vi "hanfei_OFDM_modulator.vi"(4 "error in (no error)":errorcluster, 5 "OFDM Parameters":T1={"FFT size (N)"=64, "Length of CP (Lc)"=8, "Null Tones"=[0, 30, 31, 32], "Training Sequence FFT size"=0, "Training Sequence Length of CP"=0, "Number of OFDM symbols (derived)"=1}, 7 "input symbols":cdb[](array[numeric])) -> (0 "error out":errorcluster, 1 "OFDM Parameters out":T1={"FFT size (N)"=64, "Length of CP (Lc)"=8, "Null Tones"=[0, 30, 31, 32], "Training Sequence FFT size"=0, "Training Sequence Length of CP"=0, "Number of OFDM symbols (derived)"=1}, 3 "output samples":cdb[](array[numeric]))   [LabVIEW 2015]
uses:
  OFDM_parameters.ctl
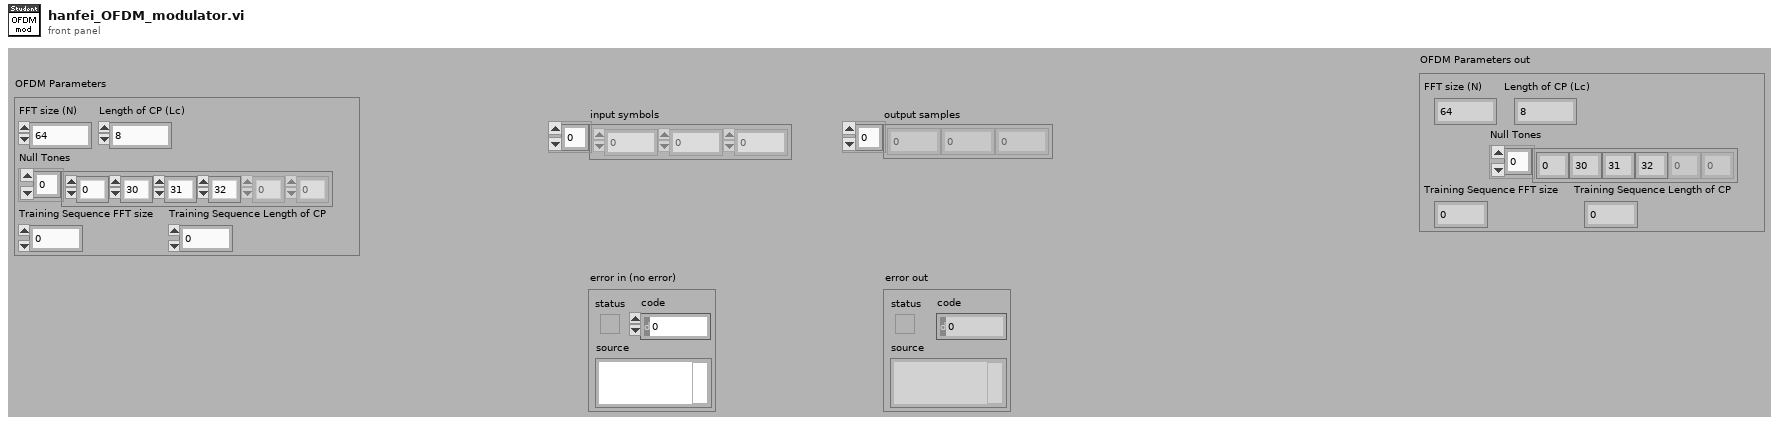
[diagram p1: front panel]
types:
  T1 = typedef "OFDM_parameters.ctl" = cluster{"FFT size (N)":i32, "Length of CP (Lc)":i32, "Null Tones":u32[], "Training Sequence FFT size":i32, "Training Sequence Length of CP":i32, "Number of OFDM symbols (derived)":i32}
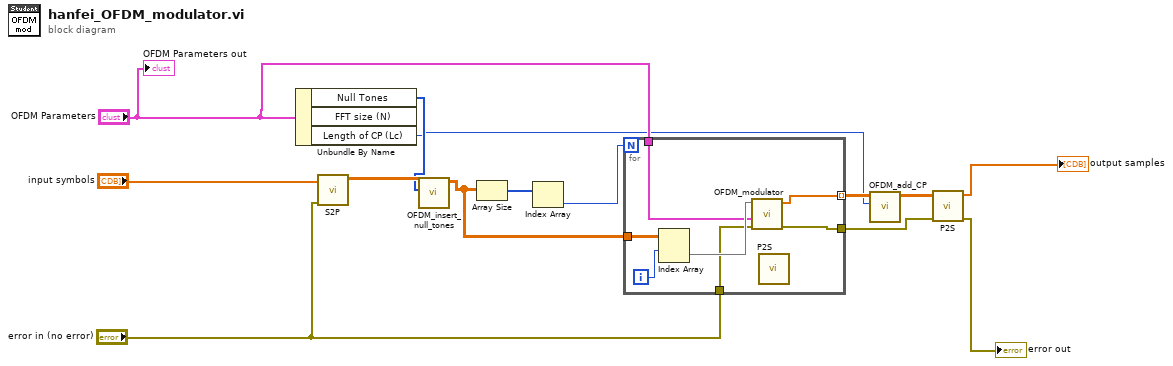
[diagram p0: block diagram]
diagram:
  n1 = Unbundle By Name("OFDM Parameters") -> ("Null Tones"=w12:u32[], "Length of CP (Lc)"=w1:i32)  [unwired: 1 out]
  n2 = call "S2P.vi"("error in (no error)"="error in (no error)", "serial input"="input symbols") -> ("parallel output"=w13:cdb[][])  [unwired: 4 in, 1 out]
  n3 = call "OFDM_insert_null_tones.vi"("null tones"=w12, "input"=w13) -> ("output"=w9:cdb[][])  [unwired: 5 in]
  n4 = Array Size(array=w9) -> (size(s)=w11:i32[])
  n5 = Index Array(array=w11) -> (element=w10:i32)  [unwired: 1 in]
  n6 = for {
    N: w10 -> [_]
    tunnel: w9 -> [w21]
    tunnel: "OFDM Parameters" -> [w18]
    tunnel: "error in (no error)" -> [w17]
    tunnel: [w16] -> w6 mode=indexing
    tunnel: [w15] -> w4
    i -> [w20]
    n7 = Index Array(array=w21, index (row)=w20) -> (element=w19:cdb[])  [unwired: 1 in]
    n8 = call "OFDM_modulator.vi"("error in (no error)"=w17, "OFDM Parameters"=w18, "input symbols"=w19) -> ("error out"=w15:errorcluster, "output samples"=w16:cdb[])  [unwired: 2 in, 1 out]
  }
  n9 = call "P2S.vi"() -> ()  [unwired: 5 in, 3 out]
  n10 = call "OFDM_add_CP.vi"("length of CP (Lc)"=w1, "input"=w6) -> ("output"=w5:cdb[][])  [unwired: 5 in]
  n11 = call "P2S.vi"("error in (no error)"=w4, "parallel input"=w5) -> ("error out"=→"error out":errorcluster, "serial output"=→"output samples":cdb[])  [unwired: 3 in, 1 out]
  "OFDM Parameters out" <- "OFDM Parameters"
